vi "GetVerticalOffset.vi"(8 "error in (no error)":errorcluster, 11 "TektronixDPO_PhysicalDevice.lvclass":refnum<class "TektronixDPO_PhysicalDevice.lvclass">) -> (0 "error out":errorcluster, 3 "TektronixDPO_PhysicalDevice.lvclassOut":refnum<class "TektronixDPO_PhysicalDevice.lvclass">)   [LabVIEW 2013, in "TektronixDPO_PhysicalDevice.lvclass"]
doc: "Read from the phsyical device the offset relative to the specified channel"
uses:
  TektronixDPO_PhysicalDevice.lvclass
  TektronixDPO_PhysicalDevice.lvclass/TektronixDPO_PhysicalDevice.ctl
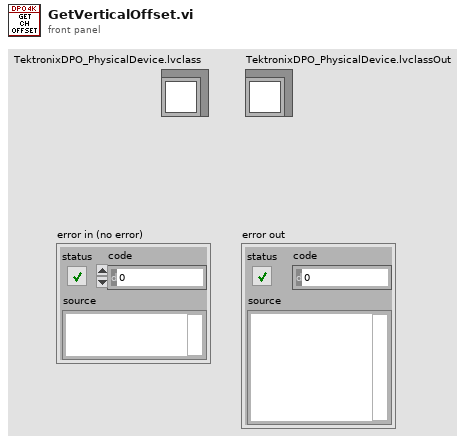
[diagram p1: front panel]
types:
  T1 = typedef "Choices.lvlib/Choice80.ctl" = u16
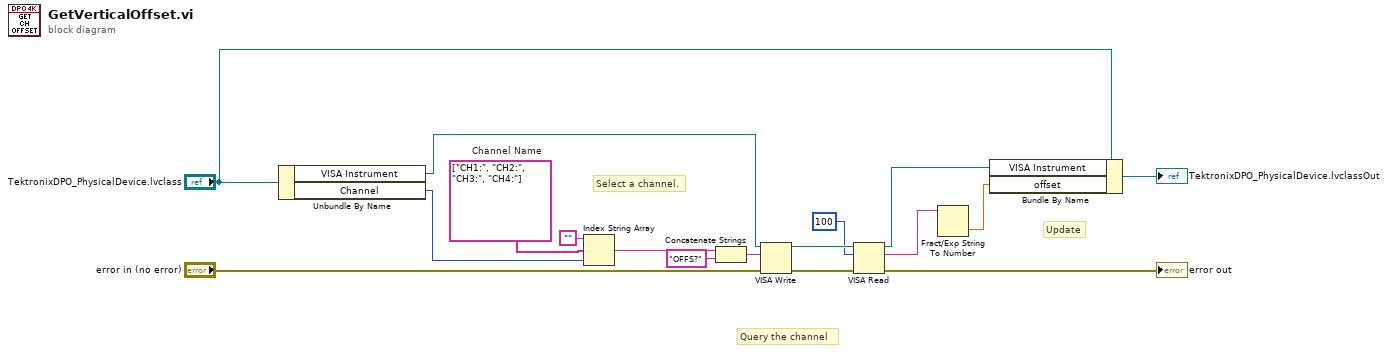
[diagram p0: block diagram]
diagram:
  w10 = string[] ["CH1:", "CH2:", "CH3:", "CH4:"]  # Channel Name
  # "Update"
  # "Query the channel"
  # "Select a channel."
  n1 = Unbundle By Name("TektronixDPO_PhysicalDevice.lvclass") -> ("VISA Instrument"=w1:refnum<visa-resource-name>, "Channel"=w4:T1)
  n2 = Index String Array(1:w4, 2:w10, 3:"") -> (0:w9:string)
  n3 = Concatenate Strings(w9, "OFFS?" ("string")) -> (w7:string)
  n4 = VISA Write(VISA resource name=w1, write buffer=w7, error in (no error)="error in (no error)") -> (VISA resource name out=w14:refnum<visa-resource-name>, error out=w12:errorcluster)  [unwired: 1 out]
  n5 = VISA Read(VISA resource name=w14, byte count=u32 100, error in (no error)=w12) -> (VISA resource name out=w3:refnum<visa-resource-name>, read buffer=w16:string, error out=→"error out":errorcluster)  [unwired: 1 out]
  n6 = Fract/Exp String To Number(string=w16) -> (number=w2:dbl)  [unwired: 3 in, 1 out]
  n7 = Bundle By Name(cluster="TektronixDPO_PhysicalDevice.lvclass", "VISA Instrument"=w3, "offset"=w2) -> (→"TektronixDPO_PhysicalDevice.lvclassOut":refnum<class "TektronixDPO_PhysicalDevice.lvclass">)
